vi "Bridge Bias Set All.vi"(8 "error in":errorcluster, 9 "Set initial biases? (False)":bool, 10 "reading":T1, 11 "bridge in":T3 {"TWM"."f-list [Hz]" format="%#_6p"}) -> (0 "error out":errorcluster, 3 "bridge out":T3 {"TWM"."f-list [Hz]" format="%#_6p"})   [LabVIEW 2013]
doc: "Set DC bias voltage of selected bias compensator channel."
uses:
  Bridge Session.ctl
  Bridge Type.ctl
  drivers/TWM client/TWM Session.ctl
  drivers/TWM client/TWM parameters.ctl
  drivers/TWM client/Meas Proc QWTB Uncertainty Mode.ctl
  Bridge Bias Session.ctl
  Bridge Bias Type.ctl
  Bridge Reading Data.ctl
  drivers/TWM client/Meas Proc QWTB Spectrum Data.ctl
  <vilib>/Utility/error.llb/Error Cluster From Error Code.vi
  <vilib>/ErrorRing/Error Ring.xnode
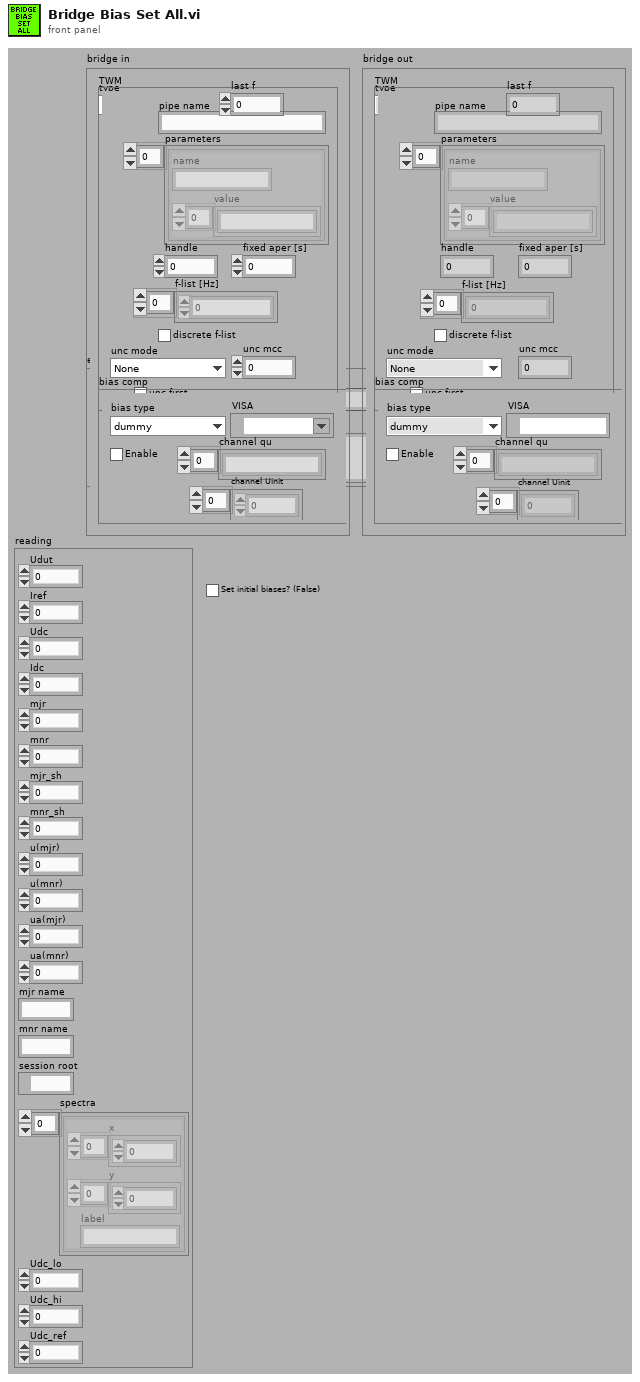
[diagram p1: front panel]
types:
  T1 = typedef "Bridge Reading Data.ctl" = cluster{"Udut":dbl, "Iref":dbl, "Udc":dbl, "Idc":dbl, "mjr":dbl, "mnr":dbl, "mjr_sh":dbl, "mnr_sh":dbl, "u(mjr)":dbl, "u(mnr)":dbl, "ua(mjr)":dbl, "ua(mnr)":dbl, "mjr name":string, "mnr name":string, "session root":path, "spectra":T2[], "Udc_lo":dbl, "Udc_hi":dbl, "Udc_ref":dbl}
  T2 = typedef "Meas Proc QWTB Spectrum Data.ctl" = cluster{"x":sgl[], "y":sgl[], "label":string}
  T3 = typedef "Bridge Session.ctl" = cluster{"type":T4, "TWM":T5, "last f":dbl, "bias comp":T8}
  T4 = typedef "Bridge Type.ctl" = enum16{"TWM client", "dummy"}
  T5 = typedef "TWM Session.ctl" = cluster{"pipe name":string, "parameters":T6[], "handle":i32, "fixed aper [s]":dbl, "f-list [Hz]":dbl[], "discrete f-list":bool, "unc mode":T7, "unc mcc":i32, "unc first":bool}
  T6 = typedef "TWM parameters.ctl" = cluster{"name":string, "value":string[]}
  T7 = typedef "Meas Proc QWTB Uncertainty Mode.ctl" = enum16{"None", "GUF", "Monte Carlo"}
  T8 = typedef "Bridge Bias Session.ctl" = cluster{"bias type":T9, "VISA":refnum<visa-resource-name>, "Enable":bool, "channel qu":string[], "channel Uinit":dbl[]}
  T9 = typedef "Bridge Bias Type.ctl" = enum16{"dummy", "CMI LiBbias V1.0"}
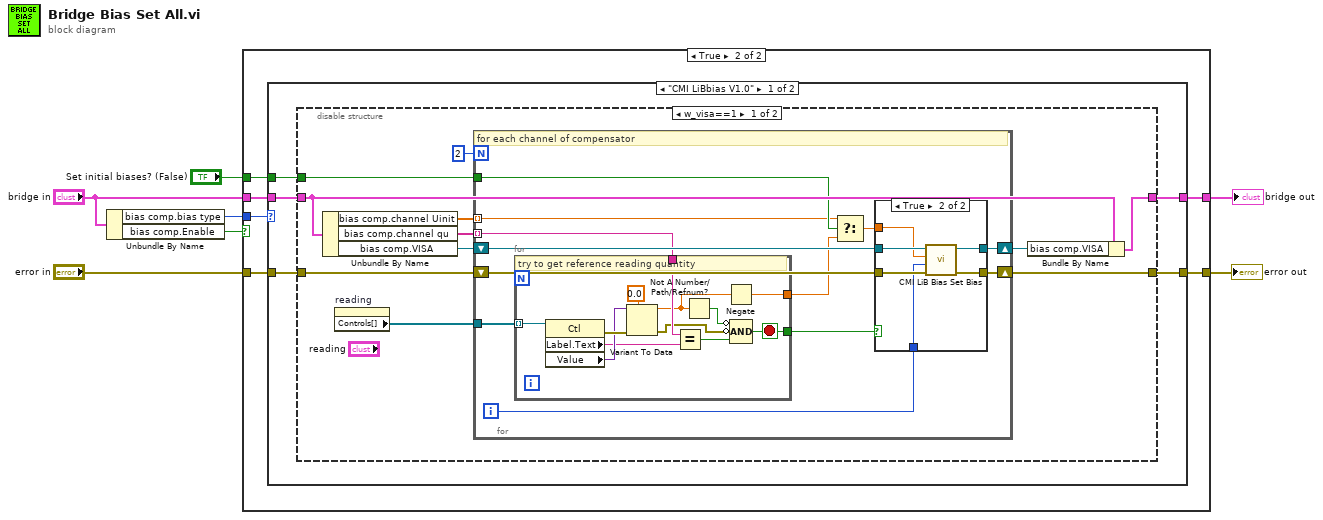
[diagram p0: block diagram]
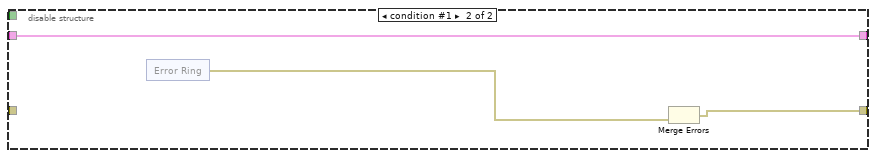
[diagram p4: hidden frame]
diagram:
  n1 = Unbundle By Name("bridge in") -> ("bias comp.bias type"=w7:T9, "bias comp.Enable"=w2:bool)
  n2 = case shown="True" w2 {
    tunnel: w7 -> [_ w15]
    tunnel: [w9 w14] -> w6
    tunnel: "bridge in" -> [w8 w13]
    tunnel: [w8 w12] -> w4
    tunnel: "error in" -> [w9 w11]
    tunnel: "Set initial biases? (False)" -> [_ w10]
    frame False {
    }
    frame True {
      n3 = case shown="\"CMI LiBbias V1.0\"" w15 {
        tunnel: [w18 w73] -> w14
        tunnel: w13 -> [w20 w74]
        tunnel: [w19 w74] -> w12
        tunnel: w11 -> [w17 w73]
        tunnel: w10 -> [w16 _]
        frame "CMI LiBbias V1.0" {
          n4 = disable-structure shown="w_visa==1" {
            disable-tunnel: w20 -> [w31 w64]
            disable-tunnel: [w30 w64] -> w19
            disable-tunnel: [w29 w65] -> w18
            disable-tunnel: w17 -> [w26 _]
            disable-tunnel: w16 -> [w22 _]
            frame condition #0 (active) {
              n5 = Unbundle By Name(w31) -> ("bias comp.channel Uinit"=w21:dbl[], "bias comp.channel qu"=w25:string[], "bias comp.VISA"=w28:refnum<visa-resource-name>)
              n6 = property on="reading" class="Clust (strict)"() -> ("Controls[]"=w24:refnum<vi>[])  [unwired: 2 in, 2 out]
              n7 = for {
                N: 2 -> [_]
                shift-right: [w41] -> w27
                shift-left: w28 -> [w42]
                shift-right: [w43] -> w29
                shift-left: w26 -> [w40]
                tunnel: w25 -> [w38] mode=indexing
                tunnel: w24 -> [w39]
                tunnel: w22 -> [w35]
                tunnel: w21 -> [w32] mode=indexing
                i -> [w36]
                # "for each channel of compensator"
                n8 = for {
                  tunnel: w39 -> [w63] mode=indexing
                  tunnel: w38 -> [w58]
                  tunnel: [w55] -> w37
                  tunnel: [w52] -> w34
                  stop <- w55 stop-if-true
                  # "try to get reference reading quantity"
                  n9 = property class="Ctl"(reference=w63) -> (error out=w62:errorcluster, "Label.Text"=w59:string, "Value"=w61:variant)  [unwired: 1 in, 1 out]
                  n10 = Variant To Data(error in=w62, type=0.0, Variant=w61) -> (data=w53:dbl, error out=w56:errorcluster)
                  n11 = Equal?(x=w58, y=w59) -> (x = y?=w57:bool)
                  n12 = Not A Number/Path/Refnum?(number/path/refnum=w53) -> (NaN/Path/Refnum?=w54:bool)
                  n13 = Negate(x=w53) -> (-x=w52:dbl)
                  n14 = Compound Arithmetic op=AND(invert w54, invert w56, w57) -> (w55:bool)
                }
                n15 = Select(t=w32, s=w35, f=w34) -> (s? t:f=w33:dbl)
                n16 = case shown="True" w37 {
                  tunnel: [w45 w51] -> w43
                  tunnel: w42 -> [w44 w50]
                  tunnel: [w44 w49] -> w41
                  tunnel: w40 -> [w45 w48]
                  tunnel: w33 -> [_ w46]
                  tunnel: w36 -> [_ w47]
                  frame False {
                  }
                  frame True {
                    n17 = call "CMI LiB Bias Set Bias.vi"("error in"=w48, "channel index (0: first)"=w47, "bias [V]"=w46, "VISA in"=w50) -> ("error out"=w51:errorcluster, "VISA out"=w49:refnum<visa-resource-name>)  [unwired: 6 in]
                  }
                }
              }
              n18 = Bundle By Name(cluster=w31, "bias comp.VISA"=w27) -> (w30:T3)
            }
            frame condition #1 {
              n19 = xnode "Error Ring"() -> ("error out"=w67:errorcluster)
              n20 = Merge Errors(w67) -> (w65:errorcluster, w66:errorcluster)
            }
          }
        }
        frame Default {
        }
      }
    }
  }
  "error out" <- w6
  "bridge out" <- w4
